vi "findStringsInArray.vi"(2 "Regular expression":string, 3 "1D string array":string[](array[string])) -> (0 "Unmatched array":string[](array[string]), 1 "Matched array":string[](array[string]))   [LabVIEW 2015]
doc: "This VI filters a 1D string array for any matches to Regular Expression and returns arrays for matching elements and unmatching elements.\n\nFunction searches each element of the 1D String Array for a pattern matching Regular Expression. The element is then appended to either the Matched Array or Unmatched Array outputs accordingly. Regular Expression can include any expression used by LabVIEW's \"Match Pattern.vi\".\n\nCurrent Version: 1.0\nLabVIEW Version: 7.1\n\nFEO Medical, Inc.\nThe PossumWorks Lab\nDeveloper: BMC"
panel:
  # "Select Help»Show Context Help and move the cursor over the VI icon to display help for this VI."
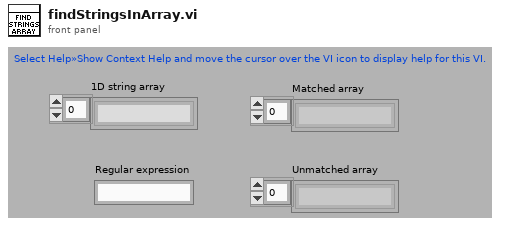
[diagram p1: front panel]
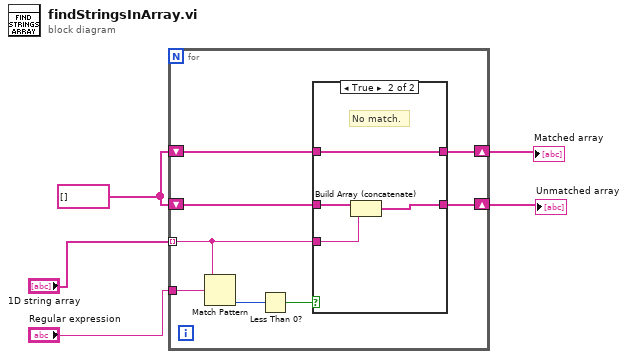
[diagram p0: block diagram]
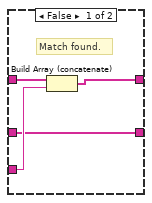
[diagram p2: hidden frame]
diagram:
  w4 = string[] []
  n1 = for {
    tunnel: "1D string array" -> [w9] mode=indexing
    tunnel: "Regular expression" -> [w13]
    shift-right: [w8] -> w2
    shift-left: w4 -> [w12]
    shift-right: [w10] -> w3
    shift-left: w4 -> [w11]
    n2 = Match Pattern(string=w9, regular expression=w13) -> (offset past match=w7:i32)  [unwired: 1 in, 3 out]
    n3 = Less Than 0?(x=w7) -> (x < 0?=w6:bool)
    n4 = case shown="True" w6 {
      tunnel: w12 -> [w15 w20]
      tunnel: w11 -> [w17 w21]
      tunnel: [w14 w21] -> w10
      tunnel: w9 -> [w16 w19]
      tunnel: [w15 w18] -> w8
      frame False {
        # "Match found."
        n5 = Build Array (concatenate)(w17, w16) -> (w14:string[])
      }
      frame True {
        # "No match."
        n6 = Build Array (concatenate)(w20, w19) -> (w18:string[])
      }
    }
  }
  "Matched array" <- w3
  "Unmatched array" <- w2
